vi "Read Sensor Servo Offset.vi"(8 "error in (no error)":errorcluster, 11 "starter kit host in":refnum<class "NI_Robotics_Starter Kit Host.lvclass">) -> (0 "error out":errorcluster, 2 "ccw offset angle (rad)":dbl, 3 "starter kit host out":refnum<class "NI_Robotics_Starter Kit Host.lvclass">)   [LabVIEW 2017, in "NI_Robotics_Starter Kit Host.lvclass"]
doc: "<B>Owning Palette:</B> Starter Kit 1.0 VIs, Starter Kit 2.0 VIs\n\nReads and returns the amount by which the zero, or straight-forward, position of the ultrasonic distance sensor is calibrated to differ from the zero position of the sensor servo."
uses:
  <vilib>/robotics/Starter Kit/Host Interface/NI_Robotics_Starter Kit Host.lvclass
  <vilib>/robotics/Starter Kit/Host Interface/NI_Robotics_Starter Kit Host.lvclass/NI_Robotics_Starter Kit Host.ctl
  <vilib>/robotics/Starter Kit/Servo Motor/NI_Robotics_Starter Kit Servo Motor.lvclass/NI_Robotics_Starter Kit Servo Motor.ctl
  <vilib>/robotics/Starter Kit/Servo Motor/NI_Robotics_Starter Kit Servo Motor.lvclass
  <vilib>/robotics/Utilities/NI_Robotics Utilities.lvlib
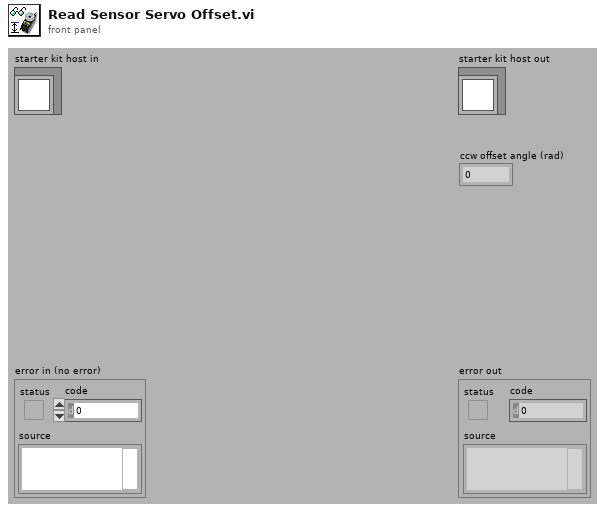
[diagram p1: front panel]
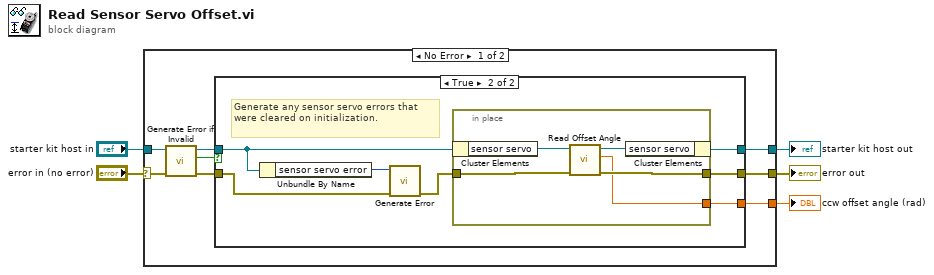
[diagram p0: block diagram]
diagram:
  n1 = case shown="No Error" "error in (no error)" {
    selector: "error in (no error)" -> [w8 w29]
    tunnel: [w12 w29] -> w3
    tunnel: [w13 w28] -> w2
    tunnel: "starter kit host in" -> [w10 w28]
    tunnel: [w11 _] -> w1
    frame No Error {
      n2 = call <vilib>:"Generate Error if Invalid.vi"("error in (no error)"=w8, "starter kit host in"=w10) -> ("error out"=w7:errorcluster, "valid?"=w6:bool, "starter kit host out"=w9:refnum<class "NI_Robotics_Starter Kit Host.lvclass">)  [unwired: 7 in]
      n3 = case shown="True" w6 {
        tunnel: [w15 w22] -> w13
        tunnel: [w14 w21] -> w12
        tunnel: [_ w20] -> w11
        tunnel: w9 -> [w15 w19]
        tunnel: w7 -> [w14 w18]
        frame False {
        }
        frame True {
          # "Generate any sensor servo errors that were cleared on initialization."
          n4 = Unbundle By Name(w19) -> ("sensor servo error"=w16:i32)
          n5 = call <vilib>:"Generate Error.vi"("error in (no error)"=w18, "code"=w16) -> ("error out"=w17:errorcluster)  [unwired: 9 in]
          n6 = in-place {
            in-place-border: w17 -> [w24]
            in-place-border: [w25] -> w21
            in-place-border: [w23] -> w20
            n7 = in-place-cluster #1(w19) -> ("sensor servo"=w27:refnum<class "NI_Robotics_Starter Kit Servo Motor.lvclass">)
            n8 = call <vilib>:"Read Offset Angle.vi"("error in (no error)"=w24, "servo motor in"=w27) -> ("error out"=w25:errorcluster, "ccw offset angle (rad)"=w23:dbl, "servo motor out"=w26:refnum<class "NI_Robotics_Starter Kit Servo Motor.lvclass">)  [unwired: 7 in]
            n9 = in-place-cluster #1("sensor servo"=w26) -> (w22:refnum<class "NI_Robotics_Starter Kit Host.lvclass">)
          }
        }
      }
    }
    frame Error {
    }
  }
  "error out" <- w3
  "starter kit host out" <- w2
  "ccw offset angle (rad)" <- w1
